vi "GetTelemetryUpdateDataConstant.vi"() -> (3 "TelemetryUpdateData":T1={"DataType"=enum."U8", "Mode"=enum."=", "Field"=enum."AnalogInputRaw4", "Data"=0})   [LabVIEW 2018]
uses:
  TelemetryUpdateData.ctl
  TelemetryDataTypes.ctl
  TelemetryUpdateModes.ctl
  TelemetryFields.ctl
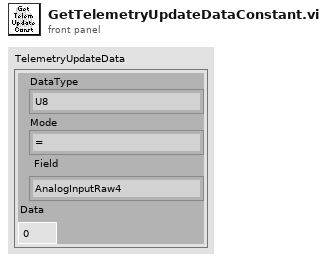
[diagram p1: front panel]
types:
  T1 = typedef "TelemetryUpdateData.ctl" = cluster{"DataType":T2, "Mode":T3, "Field":T4, "Data":u64}
  T2 = typedef "TelemetryDataTypes.ctl" = enum8{"U8", "U16", "U32", "U64", "I8", "I16", "I32", "I64", "SGL"}
  T3 = typedef "TelemetryUpdateModes.ctl" = enum8{"=", "+", "-", "|"}
  T4 = typedef "TelemetryFields.ctl" = enum16{"None", "AnalogInputSampleCount", "AnalogInputSampleTimestamp", "AnalogInputRaw1", "AnalogInputRaw2", "AnalogInputRaw3", "AnalogInputRaw4", "AnalogInputRaw5", "AnalogInputRaw6", "AnalogInputRaw7", "AnalogInputRaw8", "AnalogInputRaw9", "AnalogInputRaw10", "AnalogInputRaw11", "AnalogInputRaw12", "AnalogInputRaw13", "AnalogInputRaw14", "AnalogInputRaw15", "AnalogInputRaw16", "DigitalInputSampleCount", "DigitalInputSampleTimestamp", "DigitalInputStates", "ThermocoupleSampleCount", "ThermocoupleSampleTimestamp", "ThermocoupleRaw1", "ThermocoupleRaw2", "ThermocoupleRaw3", "ThermocoupleRaw4", "ThermocoupleRaw5", "ThermocoupleRaw6", "ThermocoupleRaw7", "ThermocoupleRaw8", "ThermocoupleRaw9", "ThermocoupleRaw10", "ThermocoupleRaw11", "ThermocoupleRaw12", "ThermocoupleRaw13", "ThermocoupleRaw14", "ThermocoupleRaw15", "ThermocoupleRaw16", "WindSensorTxBytes", "WindSensorTxFrames", "WindSensorRxBytes", "WindSensorRxFrames", "WindSensorErrorTimestamp", "WindSensorErrorCode", "WindSensorSampleTimestamp", "WindSensorXRaw", "WindSensorYRaw", "WindSensorZRaw", "WindSensorSonicTempRaw", "WindSensorDiagWord", "WindSensorRecordCount", "FlowSensorTxBytes", "FlowSensorTxFrames", "FlowSensorRxBytes", "FlowSensorRxFrames", "FlowSensorErrorTimestamp", "FlowSensorErrorCode", "FlowSensorSampleTimestamp", "FlowSensorSignalStrength", "FlowSensorFlowRate", "FlowSensorNetTotalizer", "FlowSensorPositiveTotalizer", "FlowSensorNegativeTotalizer", "FlowSensorTemperature1", "FlowSensorTemperature2", "VFDTxBytes", "VFDTxFrames", "VFDRxBytes", "VFDRxFrames", "VFDErrorTimestamp", "VFDErrorCode", "VFDSampleTimestamp", "VFDVelocityBits", "VFDDiagnosticCode", "VFDFrequencyCommand", "VFDOutputFrequency", "VFDOutputCurrent", "VFDDCBusVoltage", "VFDOutputVoltage"}
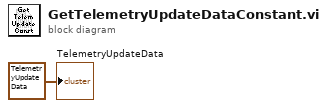
[diagram p0: block diagram]
diagram:
  "TelemetryUpdateData" <- T1 {"DataType"=enum."U8", "Mode"=enum."=", "Field"=enum."AnalogInputRaw4", "Data"=0} ("TelemetryUpdateData")
